vi "Write Binary Config.vi"(4 "Include Class Name":bool, 6 "byte order (0:big-endian, network order)":T1(ring), 8 "error in (no error)":errorcluster, 11 "StringLen_I32 in":refnum<class "StringLen_I32.lvclass">) -> (0 "error out":errorcluster, 2 "Binary":string, 3 "StringLen_I32 out":refnum<class "StringLen_I32.lvclass">)   [LabVIEW 2021, in "StringLen_I32.lvclass"]
uses:
  StringLen_I32.lvclass
  StringLen_I32.lvclass/StringLen_I32.ctl
  Abs_Types/I32 Integer/Abs_I32 Integer.lvclass
  Abs_Types/String/Abs_String.lvclass
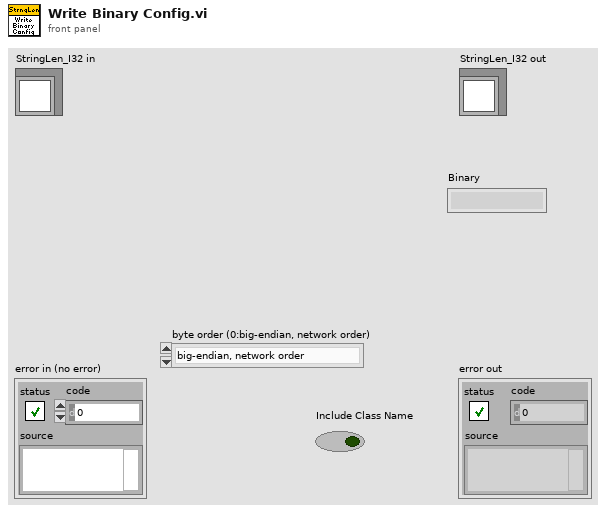
[diagram p1: front panel]
types:
  T1 = enum16{"big-endian, network order", "native, host order", "little-endian"}
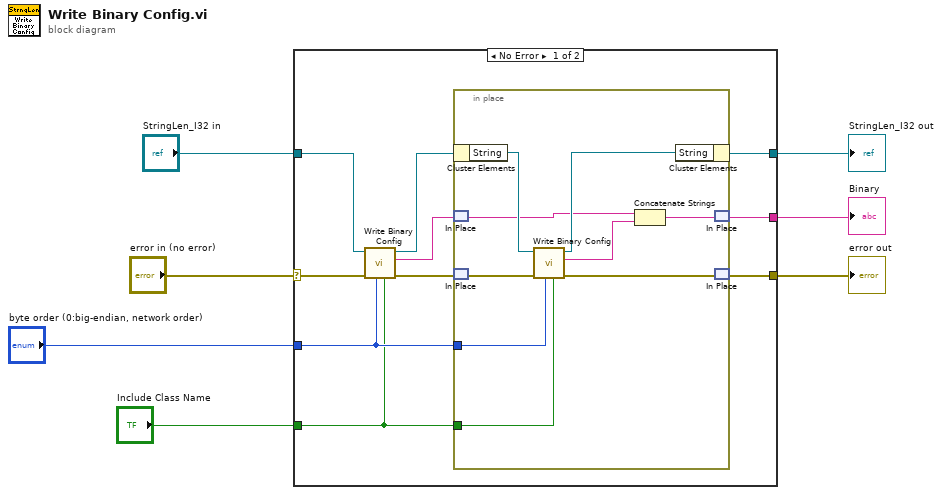
[diagram p0: block diagram]
diagram:
  n1 = case shown="No Error" "error in (no error)" {
    selector: "error in (no error)" -> [w17 w27]
    tunnel: "StringLen_I32 in" -> [w16 w28]
    tunnel: [w12 _] -> w3
    tunnel: "byte order (0:big-endian, network order)" -> [w11 _]
    tunnel: "Include Class Name" -> [w10 _]
    tunnel: [w9 w27] -> w6
    tunnel: [w8 w28] -> w4
    frame No Error {
      n2 = call-parent "Write Binary Config.vi"("Include Class Name"=w10, "byte order (0:big-endian, network order)"=w11, "error in (no error)"=w17, "Abs_Type in"=w16) -> ("error out"=w14:errorcluster, "Binary"=w13:string, "Abs_Type out"=w15:refnum<class "StringLen_I32.lvclass">)  [unwired: 5 in]
      n3 = in-place {
        in-place-border: w11 -> [w21]
        in-place-border: w10 -> [w23]
        n4 = in-place-cluster #1(w15) -> ("String"=w24:refnum<class "Abs_String.lvclass">)
        n5 = in-place-match #2(w13) -> (w20:string)
        n6 = in-place-match #3(w14) -> (w26:errorcluster)
        n7 = call-dynamic "Write Binary Config.vi"("Include Class Name"=w23, "byte order (0:big-endian, network order)"=w21, "error in (no error)"=w26, "Abs_Type in"=w24) -> ("error out"=w22:errorcluster, "Binary"=w19:string, "Abs_Type out"=w25:refnum<class "Abs_String.lvclass">)  [unwired: 5 in]
        n8 = Concatenate Strings(w20, w19) -> (w18:string)
        n9 = in-place-cluster #1("String"=w25) -> (w8:refnum<class "StringLen_I32.lvclass">)
        n10 = in-place-match #2(w18) -> (w12:string)
        n11 = in-place-match #3(w22) -> (w9:errorcluster)
      }
    }
    frame Error {
    }
  }
  "error out" <- w6
  "StringLen_I32 out" <- w4
  "Binary" <- w3
